vi "Collect Channel Snapshot Data.vi"(6 "Template waveform":waveform(dbl), 8 "error in":errorcluster, 9 "Channel Name":string, 10 "Channel":i32, 11 "3300 in":refnum<class "3300.lvclass">) -> (0 "error out":errorcluster, 2 "Channel Data":waveform(dbl)[](array[waveform]), 3 "3300 out":refnum<class "3300.lvclass">)   [LabVIEW 2019, in "3300.lvlib" / "3300.lvclass"]
uses:
  Library/3300.lvclass
  builds/Instruments/Instruments.lvlibp/Library/Instruments.lvclass
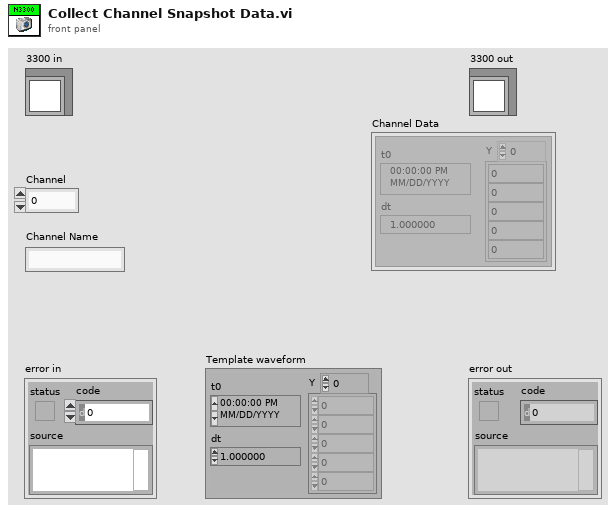
[diagram p1: front panel]
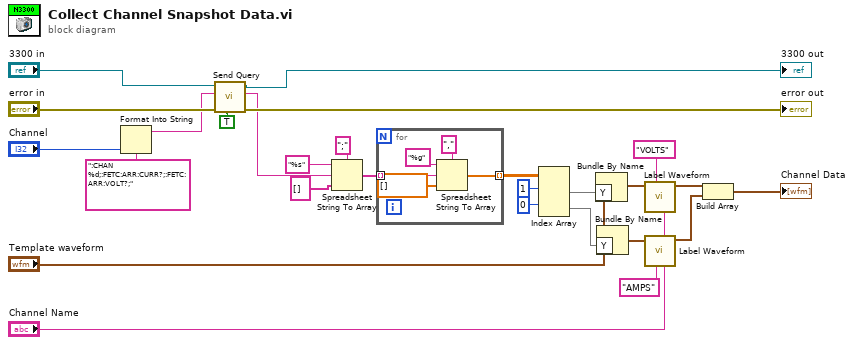
[diagram p0: block diagram]
diagram:
  n1 = Format Into String(format string=":CHAN %d;:FETC:ARR:CURR?;:FETC:ARR:VOLT?;", "Channel") -> (resulting string=w5:string)  [unwired: 2 in, 1 out]
  n2 = call "Send Query.vi"("Big Data?"=TRUE, "error in"="error in", "Query"=w5, "3300 in"="3300 in") -> ("error out"=→"error out":errorcluster, "Read Data"=w1:string, "3300 out"=→"3300 out":refnum<class "3300.lvclass">)  [unwired: 5 in]
  n3 = Spreadsheet String To Array(delimiter (Tab)=";" ("delimiter"), format string="%s", spreadsheet string=w1, array type (2D Dbl)=string[] []) -> (array=w24:string[])
  n4 = for {
    tunnel: w24 -> [w32] mode=indexing
    tunnel: [w28] -> w25 mode=indexing
    n5 = Spreadsheet String To Array(delimiter (Tab)=",", format string="%g", spreadsheet string=w32, array type (2D Dbl)=dbl[] []) -> (array=w28:dbl[])
  }
  n6 = Index Array(array=w25, index (row) #1=1 ("index (row)"), index (row) #2=0 ("index (row)")) -> (element #1=w18:dbl[], element #2=w17:dbl[])  [unwired: 2 in]
  n7 = Bundle By Name(cluster="Template waveform", "Y"=w18) -> (w15:waveform(dbl))
  n8 = Bundle By Name(cluster="Template waveform", "Y"=w17) -> (w14:waveform(dbl))
  n9 = call "Label Waveform.vi"("Unique Channel Name"="Channel Name", "Measurement"="VOLTS", "Input waveform"=w15) -> ("Labelled Waveform"=w12:waveform(dbl))  [unwired: 8 in]
  n10 = call "Label Waveform.vi"("Unique Channel Name"="Channel Name", "Measurement"="AMPS", "Input waveform"=w14) -> ("Labelled Waveform"=w13:waveform(dbl))  [unwired: 8 in]
  n11 = Build Array(w12, w13) -> (→"Channel Data":waveform(dbl)[])
